vi "Launch Task.vi"(8 "error in (no error)":errorcluster, 10 "Task":refnum<class "Task.lvclass">, 11 "VolatusCore in":refnum<class "VolatusCore.lvclass">) -> (0 "error out":errorcluster, 2 "EnQr":refnum<class "Message Enqueuer.lvclass">, 3 "VolatusCore out":refnum<class "VolatusCore.lvclass">)   [LabVIEW 2020, in "Volatus.lvlib" / "VolatusCore.lvclass"]
uses:
  VolatusCore.lvclass
  C:/Program Files (x86)/National Instruments/LabVIEW 2020/vi.lib/ActorFramework/Actor/Actor.lvclass
  Task/Task.lvclass
  <vilib>/ActorFramework/Message Enqueuer/Message Enqueuer.lvclass
  Task/Node Info.ctl
  VolatusCore.lvclass/VolatusCore.ctl
  lv-vecto/Vecto/Vecto/Vecto.lvclass/Vecto.ctl
  Task/Task.lvclass/Task.ctl
  <vilib>/ActorFramework/Actor/Actor.lvclass
  lv-vecto/Vecto/Vecto/Vecto.lvclass
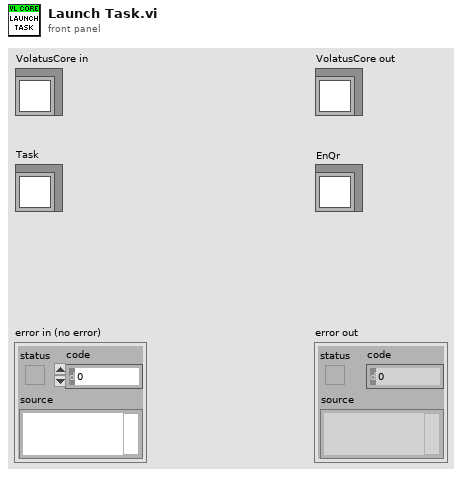
[diagram p1: front panel]
types:
  T1 = typedef "Volatus.lvlib/Task.lvclass/Node Info.ctl" = cluster{"System":string, "Cluster":string, "Node":string}
  T2 = typedef "Volatus.lvlib/Core APIs.ctl" = cluster{"Volatus":refnum<class "VolatusAPI.lvclass">, "Event":refnum<class "EventAPI.lvclass">, "Config":refnum<class "ConfigAPI.lvclass">}
  T3 = typedef "Vecto.lvlib/Node Config.lvclass/Node Info.ctl" = cluster{"System":string, "Cluster":string, "Name":string, "ID":u32, "Capabilities":string[]}
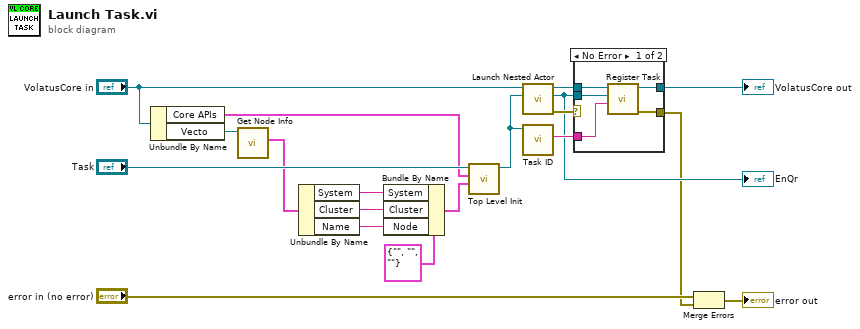
[diagram p0: block diagram]
diagram:
  n1 = Unbundle By Name("VolatusCore in") -> ("Core APIs"=w17:T2, "Vecto"=w13:refnum<class "Vecto.lvclass">)
  n2 = call "Get Node Info.vi"("Vecto in"=w13) -> ("Info"=w12:T3)  [unwired: 8 in, 2 out]
  n3 = Unbundle By Name(w12) -> ("System"=w11:string, "Cluster"=w10:string, "Name"=w9:string)
  n4 = Bundle By Name(cluster=T1 {"System"="", "Cluster"="", "Node"=""} ("Node Info"), "System"=w11, "Cluster"=w10, "Node"=w9) -> (w14:T1)
  n5 = call "Top Level Init.vi"("Node Info"=w14, "Core APIs"=w17, "Task in"="Task") -> ("Task out"=w8:refnum<class "Task.lvclass">)  [unwired: 7 in, 1 out]
  n6 = call <vilib>:"Launch Nested Actor.vi"("Nested Actor"=w8, "Caller Actor in"="VolatusCore in") -> ("error out"=w7:errorcluster, "Nested Actor's Enqueuer"=w4:refnum<class "Message Enqueuer.lvclass">, "Caller Actor out"=w6:refnum<class "VolatusCore.lvclass">)  [unwired: 7 in]
  "EnQr" <- w4
  n7 = call "Task ID.vi"("Task in"=w8) -> ("Task ID"=w5:string)  [unwired: 8 in, 2 out]
  n8 = case shown="No Error" w7 {
    selector: w7 -> [_ w25]
    tunnel: w6 -> [w24 w26]
    tunnel: w5 -> [w22 _]
    tunnel: w4 -> [w23 _]
    tunnel: [w21 w26] -> w3
    tunnel: [w20 w25] -> w1
    frame No Error {
      n9 = call "Register Task.vi"("Task ID"=w22, "EnQr"=w23, "VolatusCore in"=w24) -> ("error out"=w20:errorcluster, "VolatusCore out"=w21:refnum<class "VolatusCore.lvclass">)  [unwired: 7 in]
    }
    frame Error {
    }
  }
  "VolatusCore out" <- w3
  n10 = Merge Errors("error in (no error)", w1) -> (→"error out":errorcluster)
